vi "set_PI_Settings.vi"(0 "Interface in":T4, 5 "VDCLinkToPower":T1={"gains"={"proportional gain"=0.0, "integral gain"=0.0}, "output range"={"output high (Inf)"=inf, "output low (-Inf)"=-inf}, "PI_state"=enum."idle", "reset"=FALSE, "manual"=0.0} {"gains"."proportional gain" step=0.125}, 7 "ID_to_VD":T1={"gains"={"proportional gain"=0.0, "integral gain"=0.0}, "output range"={"output high (Inf)"=inf, "output low (-Inf)"=-inf}, "PI_state"=enum."idle", "reset"=FALSE, "manual"=0.0} {"gains"."proportional gain" step=0.125}, 9 "IQ_to_VQ":T1={"gains"={"proportional gain"=0.0, "integral gain"=0.0}, "output range"={"output high (Inf)"=inf, "output low (-Inf)"=-inf}, "PI_state"=enum."idle", "reset"=FALSE, "manual"=0.0} {"gains"."proportional gain" step=0.125}, 11 "error in":errorcluster) -> (4 "Interface out":T4, 15 "error out":errorcluster)   [LabVIEW 2017, in "AFE_interface.lvlib"]
uses:
  AFE_interface.lvlib
  InterfaceRef.ctl
  <instrlib>/_niInstr/Instruction Framework/v1/Host/Instruction Target/niInstr Instruction Target v1 Host.lvclass
  <instrlib>/_niInstr/Instruction Framework/v1/Host/Instruction Framework Context/niInstr Instruction Framework Context v1 Host.lvclass
  AFE/PI_Settings.ctl
  <vilib>/rvi/Analysis/control/PID/Typedef/niFpgaPID_PIGains.ctl
  <vilib>/rvi/Analysis/control/PID/Typedef/niFpgaPID_OutputRange.ctl
  AFE/ActiveFrontEnd.lvlib
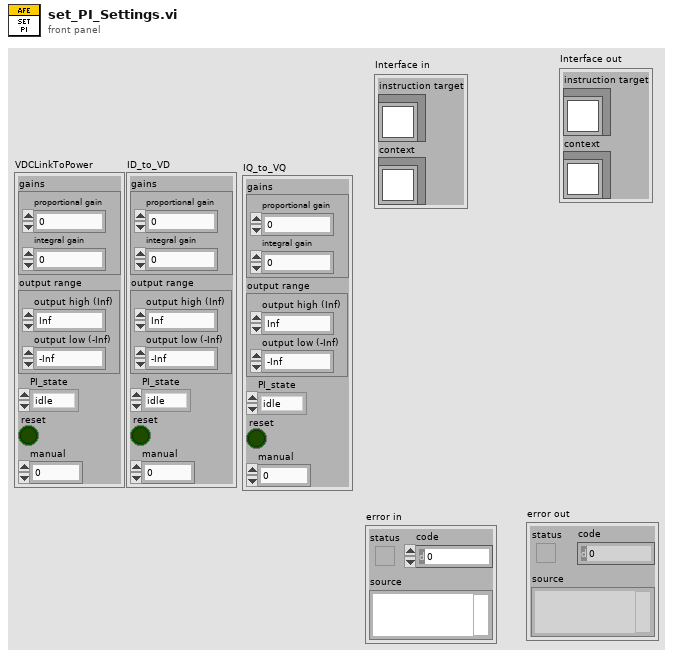
[diagram p1: front panel]
types:
  T1 = typedef "ActiveFrontEnd.lvlib/PI_Settings.ctl" = cluster{"gains":T2, "output range":T3, "PI_state":enum8{"idle", "normal", "manual", "perturbance"}, "reset":bool, "manual":sgl}
  T2 = typedef "niFpgaPID_PIGains.ctl" = cluster{"proportional gain":sgl, "integral gain":sgl}
  T3 = typedef "niFpgaPID_OutputRange.ctl" = cluster{"output high (Inf)":sgl, "output low (-Inf)":sgl}
  T4 = typedef "AFE_interface.lvlib/InterfaceRef.ctl" = cluster{"instruction target":refnum<class "niInstr Instruction Target v1 Host.lvclass">, "context":refnum<class "niInstr Instruction Framework Context v1 Host.lvclass">}
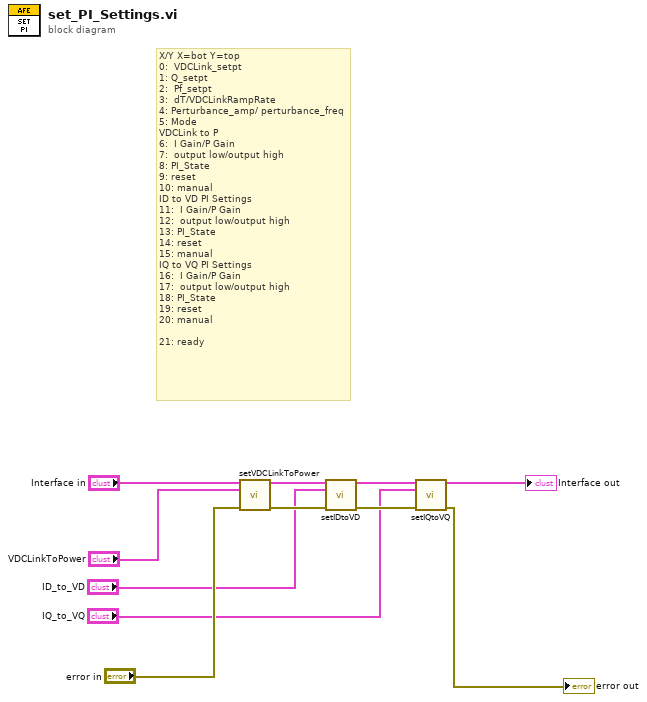
[diagram p0: block diagram]
diagram:
  # "X/Y X=bot Y=top\n0:  VDCLink_setpt\n1: Q_setpt\n2:  Pf_setpt\n3:  dT/VDCLinkRampRate\n4: Perturbance_amp/ perturbance_freq\n5: Mode\nVDCLink to P\n6:  I Gain/P Gain\n7:  output low/output high\n8: PI_State\n9: reset\n10: manual\nID to VD PI Settings \n11:  I Gain/P Gain\n12:  output low/output high\n13: PI_State\n14: reset\n15: manual\nIQ to VQ PI Settings\n16:  I Gain/P Gain\n17:  output low/output high\n18: PI_State\n19: reset\n20: manual\n\n21: ready"
  n1 = call "setVDCLinkToPower.vi"("Interface in"="Interface in", "VDCLinkToPower"="VDCLinkToPower", "error in"="error in") -> ("Interface out"=w10:T4, "error out"=w6:errorcluster)  [unwired: 11 in]
  n2 = call "setIDtoVD.vi"("Interface in"=w10, "IDtoVD"="ID_to_VD", "error in"=w6) -> ("Interface out"=w9:T4, "error out"=w5:errorcluster)  [unwired: 11 in]
  n3 = call "setIQtoVQ.vi"("Interface in"=w9, "IQtoVQ"="IQ_to_VQ", "error in"=w5) -> ("Interface out"=→"Interface out":T4, "error out"=→"error out":errorcluster)  [unwired: 11 in]
